vi "Next Rune.vi"(8 "error in (no error)":errorcluster, 11 "UTF8 in":refnum<class "UTF-8 String.lvclass">) -> (0 "error out":errorcluster, 2 "Rune":u32, 3 "UTF8 out":refnum<class "UTF-8 String.lvclass">)   [LabVIEW 2019, in "JKI Unicode.lvlib" / "UTF-8 String.lvclass"]
doc: "JKI Unicode 1.0.0.7\nTomi Maila - JKI\nCopyright (c) 2016, JKI"
uses:
  UTF-8 String.lvclass
  UTF-8 String.lvclass/UTF-8 String.ctl
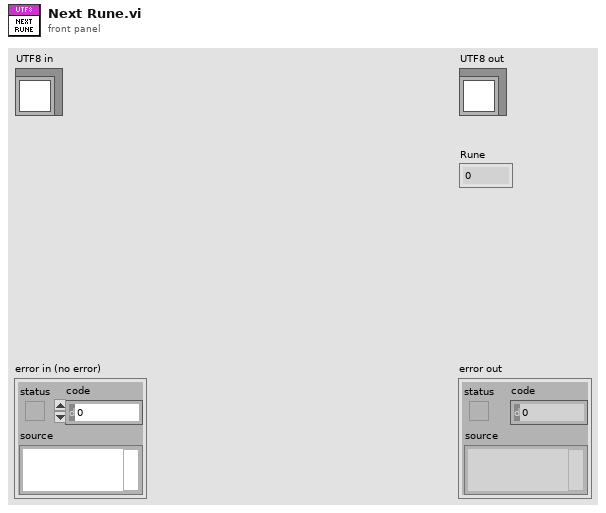
[diagram p1: front panel]
types:
  T1 = typedef "JKI Unicode.lvlib/UTF-8 String.lvclass/Byte Stream.ctl" = u8[]
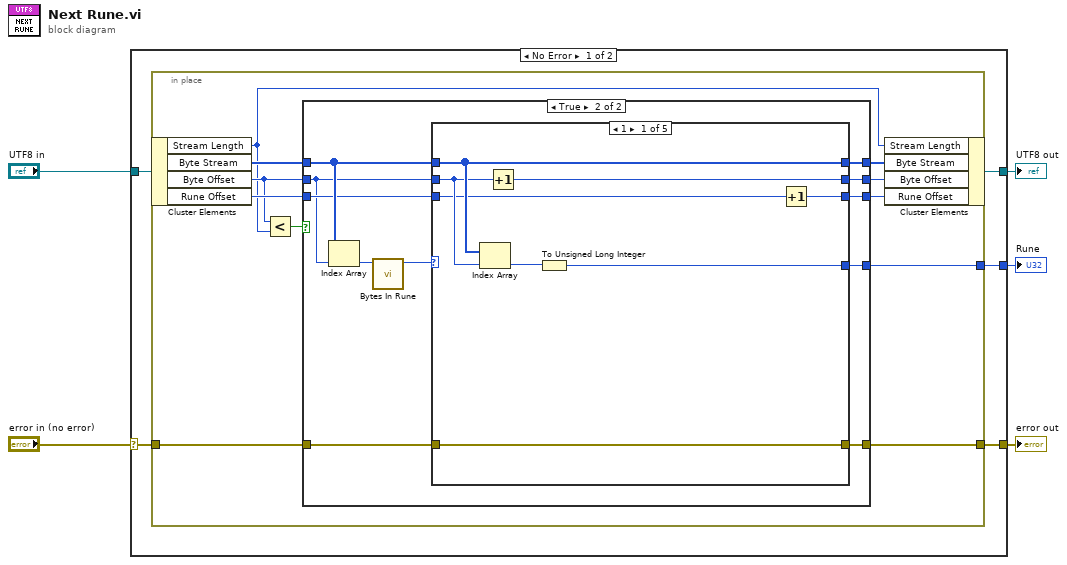
[diagram p0: block diagram]
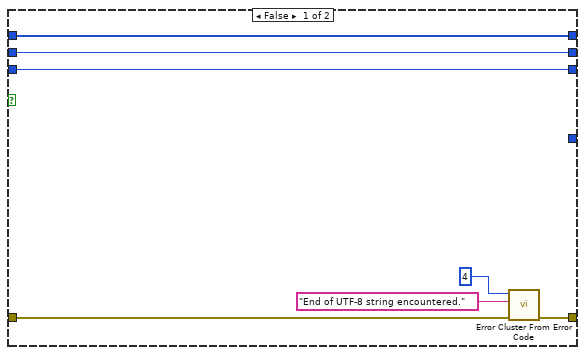
[diagram p2: hidden frame]
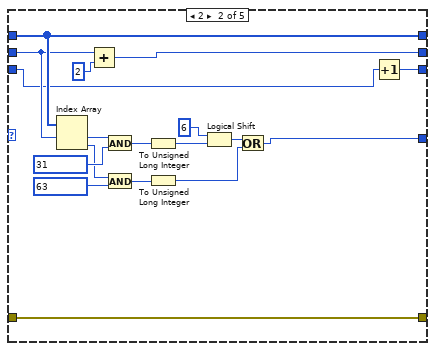
[diagram p3: hidden frame]
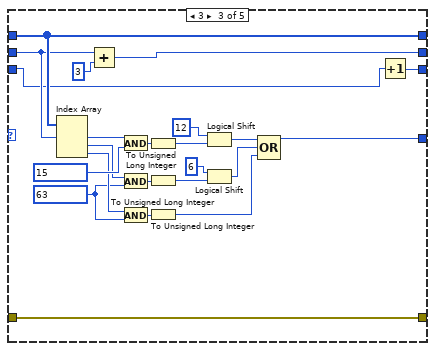
[diagram p4: hidden frame]
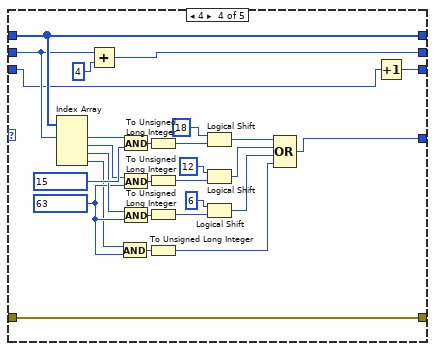
[diagram p5: hidden frame]
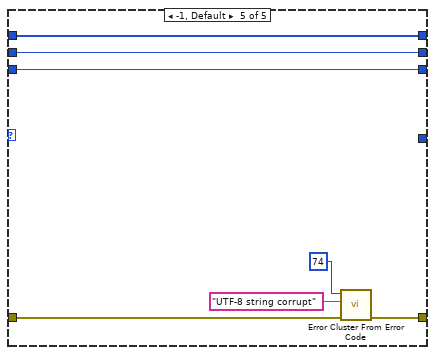
[diagram p6: hidden frame]
diagram:
  n1 = case shown="No Error" "error in (no error)" {
    selector: "error in (no error)" -> [w8 w125]
    tunnel: [w6 w125] -> w4
    tunnel: [w9 w124] -> w2
    tunnel: "UTF8 in" -> [w10 w124]
    tunnel: [w7 _] -> w1
    frame No Error {
      n2 = in-place {
        in-place-border: w8 -> [w16]
        in-place-border: [w18] -> w7
        in-place-border: [w15] -> w6
        n3 = in-place-cluster #1(w10) -> ("Stream Length"=w12:i32, "Byte Stream"=w21:T1, "Byte Offset"=w13:i32, "Rune Offset"=w17:i32)
        n4 = Less?(x=w13, y=w12) -> (x < y?=w11:bool)
        n5 = case shown="True" w11 {
          tunnel: w21 -> [w28 w37]
          tunnel: [w28 w36] -> w20
          tunnel: [w27 w35] -> w19
          tunnel: [_ w34] -> w18
          tunnel: w17 -> [w26 w33]
          tunnel: w16 -> [w24 w32]
          tunnel: [w25 w31] -> w15
          tunnel: [w26 w30] -> w14
          tunnel: w13 -> [w27 w29]
          frame False {
            n6 = call <vilib>:"Error Cluster From Error Code.vi"("error in (no error)"=w24, "error message (\"\")"="End of UTF-8 string encountered." ("error message (\"\")"), "error code (0)"=4) -> ("error out"=w25:errorcluster)  [unwired: 6 in]
          }
          frame True {
            n7 = Index Array(array=w37, index=w29) -> (element=w39:u8)
            n8 = call "Bytes In Rune.vi"("Byte"=w39) -> ("Bytes in Rune"=w38:i8)  [unwired: 10 in]
            n9 = case shown="1" w38 {
              tunnel: w37 -> [w47 w65 w88 w116 w123]
              tunnel: [w47 w65 w88 w116 w123] -> w36
              tunnel: w29 -> [w44 w63 w86 w114 w122]
              tunnel: [w45 w51 w77 w105 _] -> w34
              tunnel: [w43 w64 w87 w115 w122] -> w35
              tunnel: w33 -> [w40 w48 w66 w89 w117]
              tunnel: w32 -> [w42 w50 w68 w91 w121]
              tunnel: [w42 w50 w68 w91 w120] -> w31
              tunnel: [w41 w49 w67 w90 w117] -> w30
              frame 1 {
                n10 = Index Array(array=w47, index=w44) -> (element=w46:u8)
                n11 = Increment(x=w44) -> (x+1=w43:i32)
                n12 = To Unsigned Long Integer(number=w46) -> (unsigned 32bit integer=w45:u32)
                n13 = Increment(x=w40) -> (x+1=w41:i32)
              }
              frame 2 {
                n14 = Index Array(array=w65, index #1=w63) -> (element #1=w61:u8, element #2=w58:u8)  [unwired: 1 in]
                n15 = Add(x=w63, y=2) -> (x+y=w64:i32)
                n16 = And(x=w61, y=u8 31 ("Byte")) -> (x .and. y?=w57:u8)
                n17 = And(x=w58, y=u8 63 ("Byte")) -> (x .and. y?=w56:u8)
                n18 = To Unsigned Long Integer(number=w57) -> (unsigned 32bit integer=w55:u32)
                n19 = To Unsigned Long Integer(number=w56) -> (unsigned 32bit integer=w52:u32)
                n20 = Logical Shift(y=i16 6, x=w55) -> (x << y=w53:u32)
                n21 = Or(x=w53, y=w52) -> (x .or. y?=w51:u32)
                n22 = Increment(x=w48) -> (x+1=w49:i32)
              }
              frame 3 {
                w73 = u8 63 ("Byte")
                n23 = Index Array(array=w88, index #1=w86) -> (element #1=w84:u8, element #2=w82:u8, element #3=w74:u8)  [unwired: 2 in]
                n24 = Add(x=w86, y=3) -> (x+y=w87:i32)
                n25 = And(x=w84, y=u8 15 ("Byte")) -> (x .and. y?=w81:u8)
                n26 = And(x=w82, y=w73) -> (x .and. y?=w75:u8)
                n27 = And(x=w74, y=w73) -> (x .and. y?=w76:u8)
                n28 = To Unsigned Long Integer(number=w81) -> (unsigned 32bit integer=w80:u32)
                n29 = To Unsigned Long Integer(number=w75) -> (unsigned 32bit integer=w72:u32)
                n30 = To Unsigned Long Integer(number=w76) -> (unsigned 32bit integer=w69:u32)
                n31 = Logical Shift(y=i16 12, x=w80) -> (x << y=w78:u32)
                n32 = Logical Shift(y=i16 6, x=w72) -> (x << y=w70:u32)
                n33 = Compound Arithmetic op=OR(w78, w70, w69) -> (w77:u32)
                n34 = Increment(x=w66) -> (x+1=w67:i32)
              }
              frame 4 {
                w97 = u8 63 ("Byte")
                n35 = Index Array(array=w116, index #1=w114) -> (element #1=w112:u8, element #2=w110:u8, element #3=w98:u8, element #4=w92:u8)  [unwired: 3 in]
                n36 = Add(x=w114, y=4) -> (x+y=w115:i32)
                n37 = And(x=w92, y=w97) -> (x .and. y?=w99:u8)
                n38 = And(x=w112, y=u8 15 ("Byte")) -> (x .and. y?=w109:u8)
                n39 = And(x=w110, y=w97) -> (x .and. y?=w103:u8)
                n40 = And(x=w98, y=w97) -> (x .and. y?=w104:u8)
                n41 = To Unsigned Long Integer(number=w109) -> (unsigned 32bit integer=w108:u32)
                n42 = To Unsigned Long Integer(number=w103) -> (unsigned 32bit integer=w102:u32)
                n43 = To Unsigned Long Integer(number=w104) -> (unsigned 32bit integer=w94:u32)
                n44 = To Unsigned Long Integer(number=w99) -> (unsigned 32bit integer=w96:u32)
                n45 = Logical Shift(y=i16 18, x=w108) -> (x << y=w106:u32)
                n46 = Logical Shift(y=i16 12, x=w102) -> (x << y=w100:u32)
                n47 = Logical Shift(y=i16 6, x=w94) -> (x << y=w93:u32)
                n48 = Compound Arithmetic op=OR(w106, w100, w93, w96) -> (w105:u32)
                n49 = Increment(x=w89) -> (x+1=w90:i32)
              }
              frame -1, Default {
                n50 = call <vilib>:"Error Cluster From Error Code.vi"("error in (no error)"=w121, "error message (\"\")"="UTF-8 string corrupt" ("error message (\"\")"), "error code (0)"=74) -> ("error out"=w120:errorcluster)  [unwired: 6 in]
              }
            }
          }
        }
        n51 = in-place-cluster #1("Stream Length"=w12, "Byte Stream"=w20, "Byte Offset"=w19, "Rune Offset"=w14) -> (w9:refnum<class "UTF-8 String.lvclass">)
      }
    }
    frame Error {
    }
  }
  "error out" <- w4
  "UTF8 out" <- w2
  "Rune" <- w1
